vi "string_to_mV_Rev_02.vi"(0 "Received HEX":string) -> (1 "Byte 0 H 2":u8, 2 "Byte 0 L 2":u8, 3 "OUT 10":dbl, 4 "OUT 9":dbl, 5 "OUT":dbl, 6 "OUT 8":dbl, 8 "OUT 7":dbl, 9 "OUT 2":dbl, 10 "Byte 0 H":u8, 11 "OUT 3":dbl, 12 "OUT 4":dbl, 13 "Byte 0 L":u8, 14 "OUT 5":dbl, 15 "OUT 6":dbl)   [LabVIEW 2012]
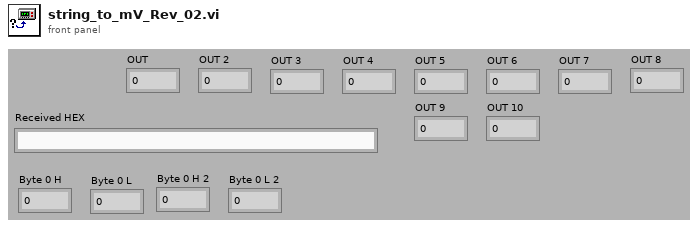
[diagram p1: front panel]
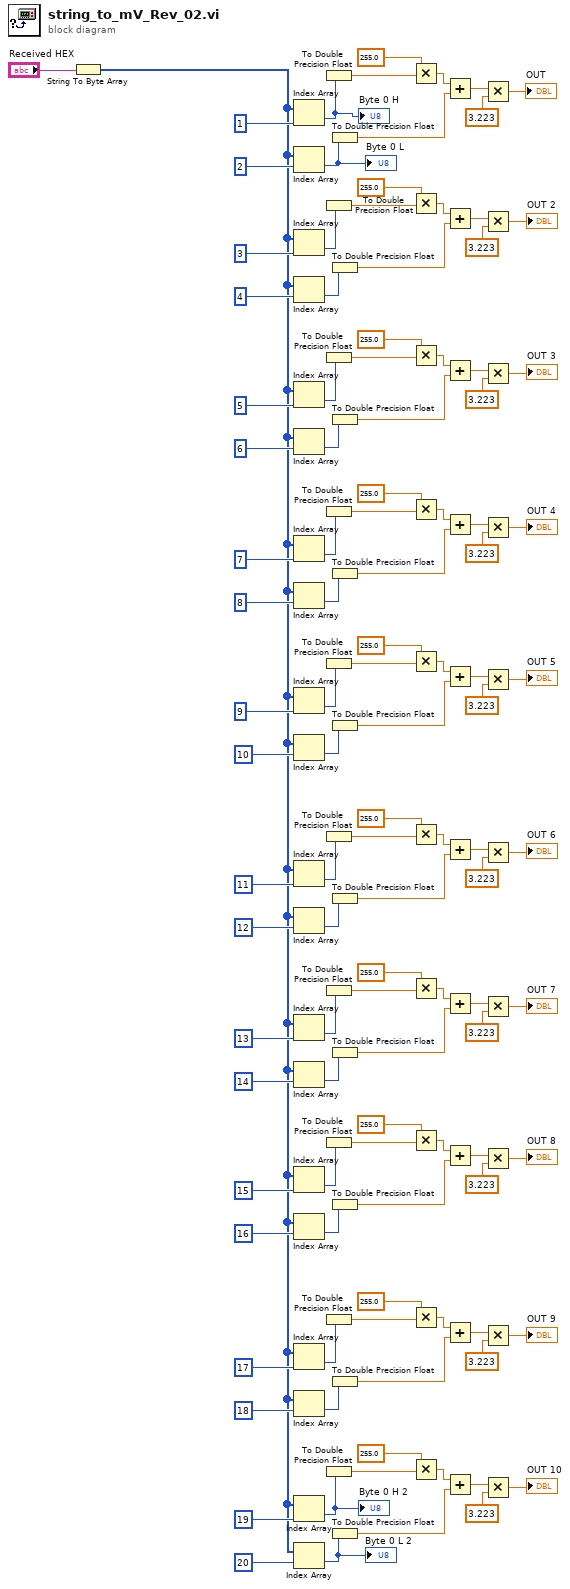
[diagram p0: block diagram]
diagram:
  n1 = String To Byte Array(string="Received HEX") -> (unsigned byte array=w5:u8[])
  n2 = Index Array(array=w5, index=1) -> (element=w4:u8)
  "Byte 0 H" <- w4
  n3 = Index Array(array=w5, index=2) -> (element=w3:u8)
  "Byte 0 L" <- w3
  n4 = Index Array(array=w5, index=3) -> (element=w103:u8)
  n5 = Index Array(array=w5, index=4) -> (element=w102:u8)
  n6 = Index Array(array=w5, index=5) -> (element=w92:u8)
  n7 = Index Array(array=w5, index=6) -> (element=w91:u8)
  n8 = Index Array(array=w5, index=7) -> (element=w80:u8)
  n9 = Index Array(array=w5, index=8) -> (element=w79:u8)
  n10 = Index Array(array=w5, index=9) -> (element=w70:u8)
  n11 = Index Array(array=w5, index=10) -> (element=w69:u8)
  n12 = Index Array(array=w5, index=11) -> (element=w58:u8)
  n13 = Index Array(array=w5, index=12) -> (element=w57:u8)
  n14 = Index Array(array=w5, index=13) -> (element=w47:u8)
  n15 = Index Array(array=w5, index=14) -> (element=w46:u8)
  n16 = Index Array(array=w5, index=15) -> (element=w37:u8)
  n17 = Index Array(array=w5, index=16) -> (element=w36:u8)
  n18 = Index Array(array=w5, index=17) -> (element=w25:u8)
  n19 = Index Array(array=w5, index=18) -> (element=w24:u8)
  n20 = Index Array(array=w5, index=19) -> (element=w2:u8)
  "Byte 0 H 2" <- w2
  n21 = Index Array(array=w5, index=20) -> (element=w1:u8)
  "Byte 0 L 2" <- w1
  n22 = To Double Precision Float(number=w4) -> (double precision float=w111:dbl)
  n23 = To Double Precision Float(number=w103) -> (double precision float=w100:dbl)
  n24 = To Double Precision Float(number=w92) -> (double precision float=w89:dbl)
  n25 = To Double Precision Float(number=w80) -> (double precision float=w77:dbl)
  n26 = To Double Precision Float(number=w70) -> (double precision float=w67:dbl)
  n27 = To Double Precision Float(number=w58) -> (double precision float=w55:dbl)
  n28 = To Double Precision Float(number=w47) -> (double precision float=w44:dbl)
  n29 = To Double Precision Float(number=w37) -> (double precision float=w34:dbl)
  n30 = To Double Precision Float(number=w25) -> (double precision float=w22:dbl)
  n31 = To Double Precision Float(number=w2) -> (double precision float=w14:dbl)
  n32 = To Double Precision Float(number=w3) -> (double precision float=w109:dbl)
  n33 = To Double Precision Float(number=w102) -> (double precision float=w98:dbl)
  n34 = To Double Precision Float(number=w91) -> (double precision float=w87:dbl)
  n35 = To Double Precision Float(number=w79) -> (double precision float=w75:dbl)
  n36 = To Double Precision Float(number=w69) -> (double precision float=w65:dbl)
  n37 = To Double Precision Float(number=w57) -> (double precision float=w53:dbl)
  n38 = To Double Precision Float(number=w46) -> (double precision float=w42:dbl)
  n39 = To Double Precision Float(number=w36) -> (double precision float=w32:dbl)
  n40 = To Double Precision Float(number=w24) -> (double precision float=w20:dbl)
  n41 = To Double Precision Float(number=w1) -> (double precision float=w12:dbl)
  n42 = Multiply(x=255.0, y=w111) -> (x*y=w110:dbl)
  n43 = Multiply(x=255.0, y=w100) -> (x*y=w99:dbl)
  n44 = Multiply(x=255.0, y=w89) -> (x*y=w88:dbl)
  n45 = Multiply(x=255.0, y=w77) -> (x*y=w76:dbl)
  n46 = Multiply(x=255.0, y=w67) -> (x*y=w66:dbl)
  n47 = Multiply(x=255.0, y=w55) -> (x*y=w54:dbl)
  n48 = Multiply(x=255.0, y=w44) -> (x*y=w43:dbl)
  n49 = Multiply(x=255.0, y=w34) -> (x*y=w33:dbl)
  n50 = Multiply(x=255.0, y=w22) -> (x*y=w21:dbl)
  n51 = Multiply(x=255.0, y=w14) -> (x*y=w13:dbl)
  n52 = Add(x=w110, y=w109) -> (x+y=w108:dbl)
  n53 = Add(x=w99, y=w98) -> (x+y=w97:dbl)
  n54 = Add(x=w88, y=w87) -> (x+y=w86:dbl)
  n55 = Add(x=w76, y=w75) -> (x+y=w74:dbl)
  n56 = Add(x=w66, y=w65) -> (x+y=w64:dbl)
  n57 = Add(x=w54, y=w53) -> (x+y=w52:dbl)
  n58 = Add(x=w43, y=w42) -> (x+y=w41:dbl)
  n59 = Add(x=w33, y=w32) -> (x+y=w31:dbl)
  n60 = Add(x=w21, y=w20) -> (x+y=w19:dbl)
  n61 = Add(x=w13, y=w12) -> (x+y=w11:dbl)
  n62 = Multiply(x=w108, y=3.223) -> (x*y=→"OUT":dbl)
  n63 = Multiply(x=w97, y=3.223) -> (x*y=→"OUT 2":dbl)
  n64 = Multiply(x=w86, y=3.223) -> (x*y=→"OUT 3":dbl)
  n65 = Multiply(x=w74, y=3.223) -> (x*y=→"OUT 4":dbl)
  n66 = Multiply(x=w64, y=3.223) -> (x*y=→"OUT 5":dbl)
  n67 = Multiply(x=w52, y=3.223) -> (x*y=→"OUT 6":dbl)
  n68 = Multiply(x=w41, y=3.223) -> (x*y=→"OUT 7":dbl)
  n69 = Multiply(x=w31, y=3.223) -> (x*y=→"OUT 8":dbl)
  n70 = Multiply(x=w19, y=3.223) -> (x*y=→"OUT 9":dbl)
  n71 = Multiply(x=w11, y=3.223) -> (x*y=→"OUT 10":dbl)
